vi "dataProcessing.vi"(2 "参考信号":dbl[](array[numeric]), 3 "中频信号":dbl[](array[numeric])) -> (0 "mean_Q":dbl, 1 "mean_I":dbl)   [LabVIEW 2018]
uses:
  <vilib>/Analysis/NI_AALPro.lvlib
panel:
  out "test2":dbl[](array[numeric])
  out "test1":dbl[](array[numeric])
  in  "sum_Q":dbl
  in  "sum_I":dbl
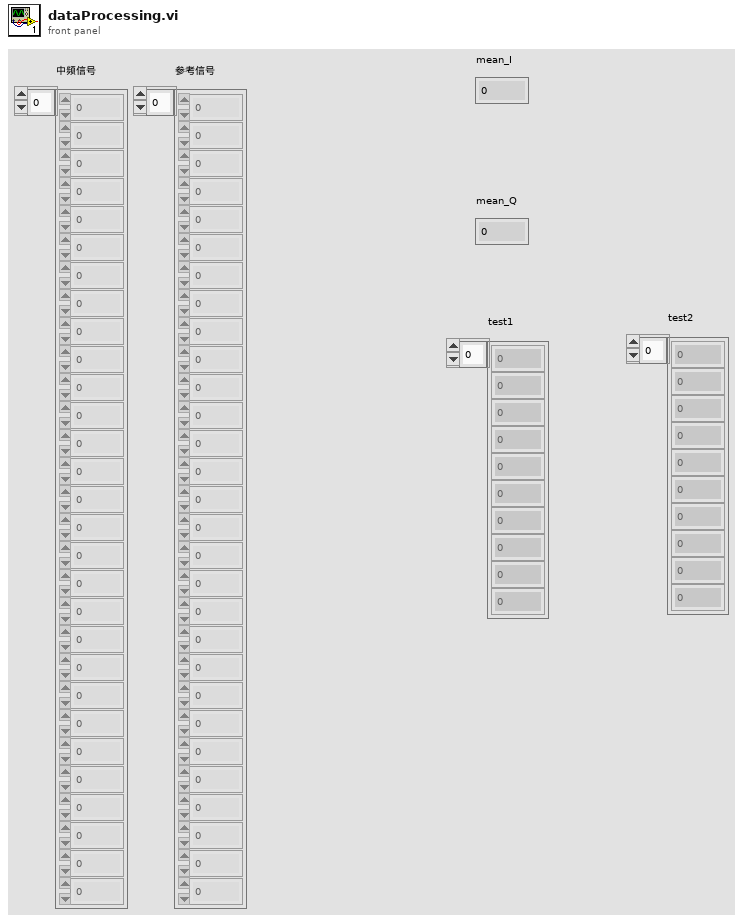
[diagram p1: front panel]
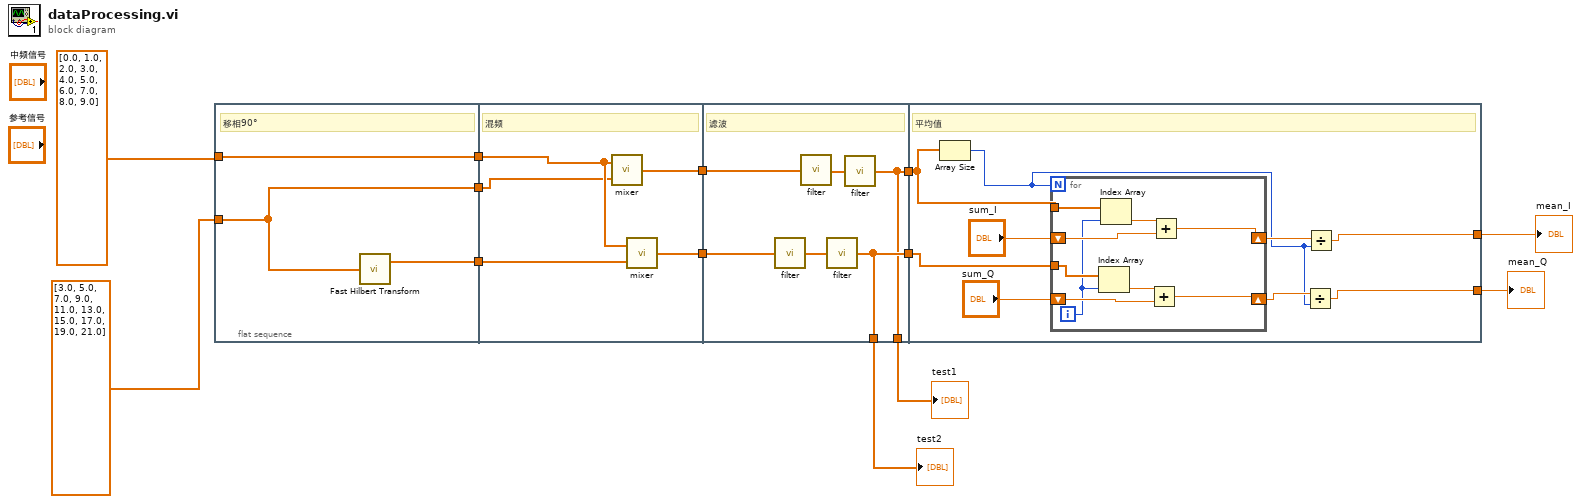
[diagram p0: block diagram]
diagram:
  n1 = flat-sequence {
    tunnel: [w15] -> w13
    tunnel: dbl[] [0.0, 1.0, 2.0, 3.0, 4.0, 5.0, 6.0, 7.0, 8.0, 9.0] -> [w15]
    tunnel: dbl[] [3.0, 5.0, 7.0, 9.0, 11.0, 13.0, 15.0, 17.0, 19.0, 21.0] -> [w14]
    tunnel: [w16] -> w10
    tunnel: [w14] -> w9
    tunnel: w13 -> [w21]
    tunnel: [w18] -> w12
    tunnel: [w17] -> w11
    tunnel: w10 -> [w19]
    tunnel: w9 -> [w20]
    tunnel: w12 -> [w27]
    tunnel: w11 -> [w25]
    tunnel: [w22] -> w8
    tunnel: [w23] -> w7
    tunnel: [w22] -> w2
    tunnel: [w23] -> w1
    tunnel: w8 -> [w33]
    tunnel: w7 -> [w34]
    tunnel: [w29] -> w6
    tunnel: [w28] -> w5
    frame #0 {
      # "移相90°"
      n2 = call <vilib>:"Fast Hilbert Transform.vi"("X"=w14) -> ("Hilbert{X}"=w16:dbl[])  [unwired: 1 out]
    }
    frame #1 {
      # "混频"
      n3 = call "mixer.vi"("参考信号"=w20, "中频信号"=w21) -> ("混频信号输出"=w18:dbl[])
      n4 = call "mixer.vi"("参考信号"=w19, "中频信号"=w21) -> ("混频信号输出"=w17:dbl[])
    }
    frame #2 {
      # "滤波"
      n5 = call "filter.vi"("输入数组"=w25) -> ("输出数组"=w24:dbl[])
      n6 = call "filter.vi"("输入数组"=w27) -> ("输出数组"=w26:dbl[])
      n7 = call "filter.vi"("输入数组"=w24) -> ("输出数组"=w23:dbl[])
      n8 = call "filter.vi"("输入数组"=w26) -> ("输出数组"=w22:dbl[])
    }
    frame #3 {
      # "平均值"
      n9 = Array Size(array=w33) -> (size(s)=w30:i32)
      n10 = for {
        N: w30 -> [_]
        tunnel: w34 -> [w39]
        tunnel: w33 -> [w44]
        shift-right: [w42] -> w32
        shift-left: "sum_I" -> [w45]
        shift-right: [w37] -> w31
        shift-left: "sum_Q" -> [w40]
        i -> [w38]
        n11 = Index Array(array=w39, index=w38) -> (element=w41:dbl)
        n12 = Index Array(array=w44, index=w38) -> (element=w43:dbl)
        n13 = Add(x=w41, y=w40) -> (x+y=w37:dbl)
        n14 = Add(x=w43, y=w45) -> (x+y=w42:dbl)
      }
      n15 = Divide(x=w31, y=w30) -> (x/y=w28:dbl)
      n16 = Divide(x=w32, y=w30) -> (x/y=w29:dbl)
    }
  }
  "mean_Q" <- w5
  "mean_I" <- w6
  "test1" <- w2
  "test2" <- w1
